vi "QTrkSetLocalizationMode.vi"(8 "Normalize profile":bool=TRUE, 9 "Z Command":T2, 10 "2D Localization Type":T3, 11 "QTrk Instance":T1) -> (3 "QTrk Instance":T1)   [LabVIEW 2011]
uses:
  QTrkInstance.ctl
  QTrkLocalizationType.ctl
  QTrkZCommandType.ctl
  QTrkDLL.vi
panel:
  out "error out":errorcluster
  in  "error in (no error)":errorcluster
  out "QTrk Instance":T1
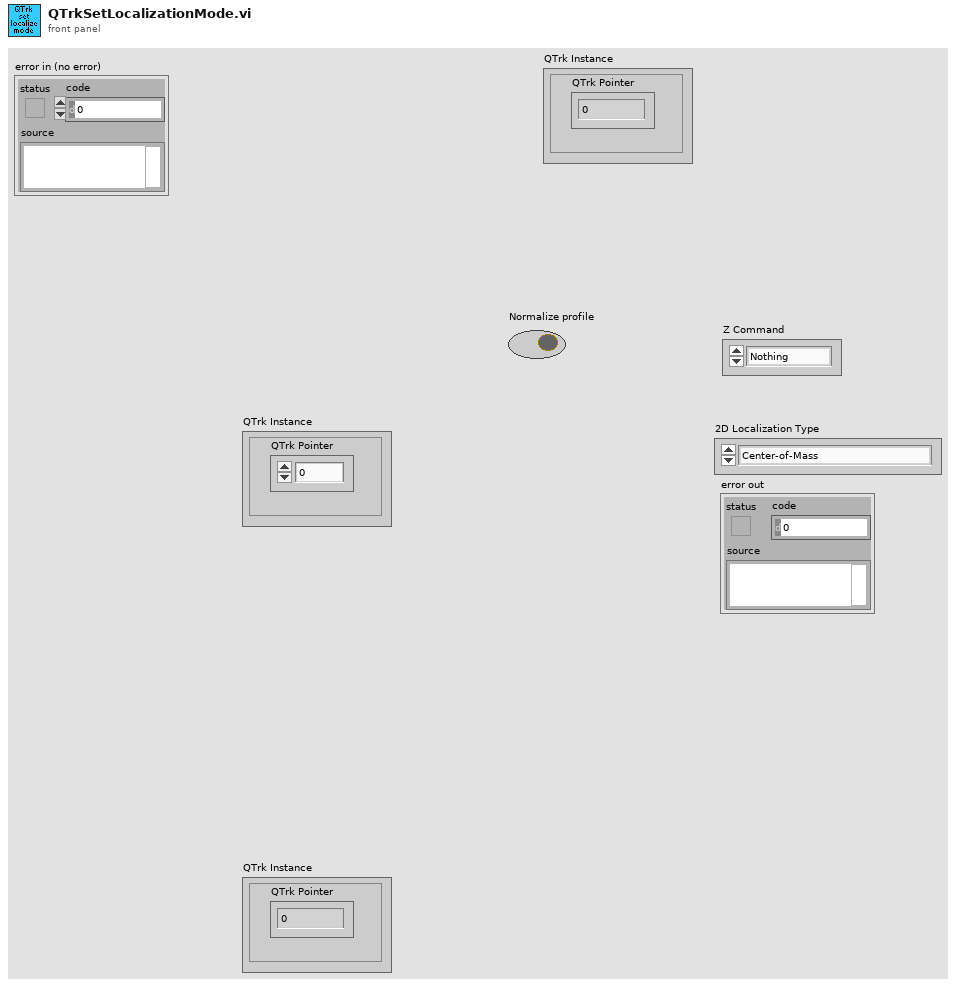
[diagram p1: front panel]
types:
  T1 = typedef "QTrkInstance.ctl" = cluster{"QTrk Pointer":u64}
  T2 = typedef "QTrkZCommandType.ctl" = enum16{"Nothing", "ComputeZ", "BuildRadialZLUT", "BuildImageZLUT", "RadialZLUT+ImageZLUT"}
  T3 = typedef "QTrkLocalizationType.ctl" = enum16{"Center-of-Mass", "1D Cross-Correlation", "Quadrant Interpolation", "Gaussian 2D MLE"}
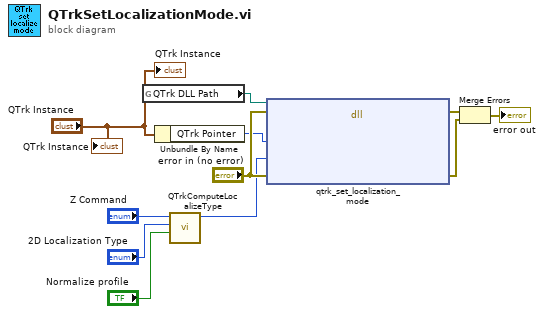
[diagram p0: block diagram]
diagram:
  n1 = global read "QTrkDLL.vi" "QTrk DLL Path"() -> (w5:path)
  n2 = Unbundle By Name("QTrk Instance") -> ("QTrk Pointer"=w6:u64)
  n3 = call "QTrkComputeLocalizeType.vi"("Normalize profile"="Normalize profile", "2D Localization Type (COM) in"="2D Localization Type", "Z Command (None)"="Z Command") -> ("Localize Type + Flags"=w1:i32)  [unwired: 8 in]
  n4 = dll-call lib="D:/jcnossen1/qtrk/qtrk/lv/qtrk-labview.dll" fn="qtrk_set_localization_mode"(path in=w5, error in="error in (no error)", "tracker"=w6, "localizeMode"=w1, "error"="error in (no error)") -> (error out=w9:errorcluster, "error"=w8:errorcluster)  [unwired: 4 in, 1 out]
  n5 = Merge Errors(w9, w8) -> (→"error out":errorcluster)
  "QTrk Instance" <- "QTrk Instance"
  "QTrk Instance" <- "QTrk Instance"
